vi "init.vi"(8 "error in (no error)":errorcluster, 11 "imaginaryStage in":refnum<class "imaginaryStage.lvclass">) -> (0 "error out":errorcluster, 3 "imaginaryStage out":refnum<class "imaginaryStage.lvclass">)   [LabVIEW 2018, in "imaginaryStage.lvclass"]
uses:
  imaginaryStage.lvclass
panel:
  in  "max pos":dbl=300.0 format="%#_13g"
  out "resource name out":string
  in  "resource name":string
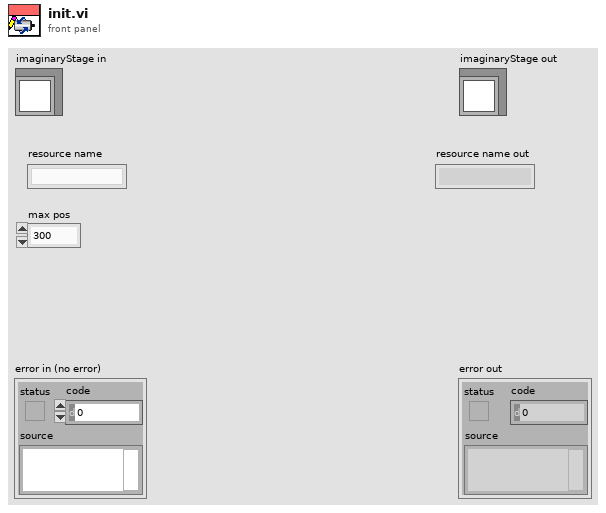
[diagram p1: front panel]
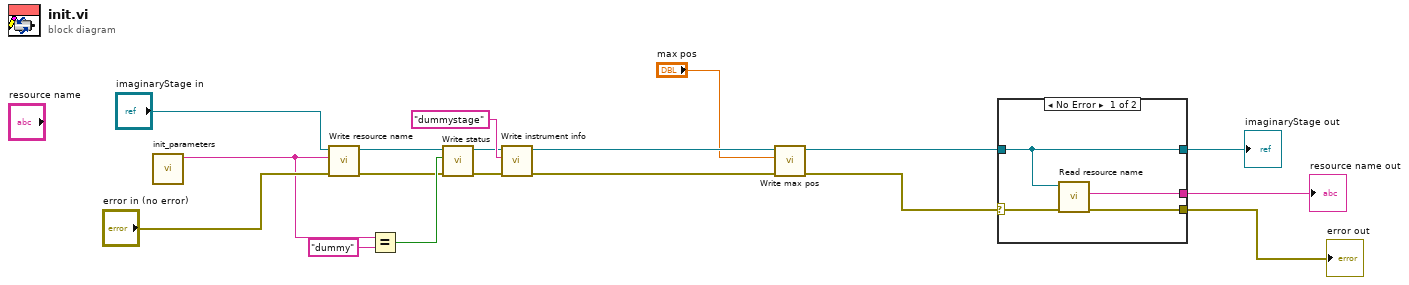
[diagram p0: block diagram]
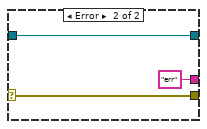
[diagram p2: hidden frame]
diagram:
  n1 = call "init_parameters.vi"() -> ("Resource name out"=w11:string)  [unwired: 11 in]
  n2 = call-dynamic "Write resource name.vi"("error in (no error)"="error in (no error)", "resource name"=w11, "_delayStageBase in"="imaginaryStage in") -> ("error out"=w7:errorcluster, "_delayStageBase out"=w12:refnum<class "imaginaryStage.lvclass">)  [unwired: 7 in]
  n3 = Equal?(x=w11, y="dummy") -> (x = y?=w9:bool)
  n4 = call-dynamic "Write status.vi"("error in (no error)"=w7, "status"=w9, "_delayStageBase in"=w12) -> ("error out"=w6:errorcluster, "_delayStageBase out"=w8:refnum<class "imaginaryStage.lvclass">)  [unwired: 7 in]
  n5 = call-dynamic "Write instrument info.vi"("error in (no error)"=w6, "instrument info"="dummystage", "_delayStageBase in"=w8) -> ("error out"=w4:errorcluster, "_delayStageBase out"=w5:refnum<class "imaginaryStage.lvclass">)  [unwired: 7 in]
  n6 = call-dynamic "Write max pos.vi"("error in (no error)"=w4, "max pos"="max pos", "_delayStageBase in"=w5) -> ("error out"=w2:errorcluster, "_delayStageBase out"=w3:refnum<class "imaginaryStage.lvclass">)  [unwired: 7 in]
  n7 = case shown="No Error" w2 {
    selector: w2 -> [w21 w25]
    tunnel: [w20 w25] -> w18
    tunnel: w3 -> [w22 w24]
    tunnel: [w22 w24] -> w17
    tunnel: [w19 "err" ("resource name")] -> w16
    frame No Error {
      n8 = call-dynamic "Read resource name.vi"("error in (no error)"=w21, "_delayStageBase in"=w22) -> ("error out"=w20:errorcluster, "resource name"=w19:string)  [unwired: 7 in, 1 out]
    }
    frame Error {
    }
  }
  "error out" <- w18
  "imaginaryStage out" <- w17
  "resource name out" <- w16
